vi "Remove Connection from State (SysDef).vi"(8 "error in (no error)":errorcluster, 9 "Connection":T1, 10 "State":string, 11 "Channel Ref in":T2 format="%.0x") -> (0 "error out":errorcluster, 1 "connection found":bool, 3 "Channel Ref out":T2=18446744073709551615 format="%.0x")   [LabVIEW 2017, in "Switch Scripting.lvlib"]
uses:
  Switch Scripting.lvlib
  <vilib>/NI Veristand/Custom Device API/Custom Device Item Ref.ctl
  Connection.ctl
  NationalInstruments.VeriStand.SystemDefinitionAPI
  <vilib>/NI VeriStand/Custom Device API/Custom Device API.lvlib
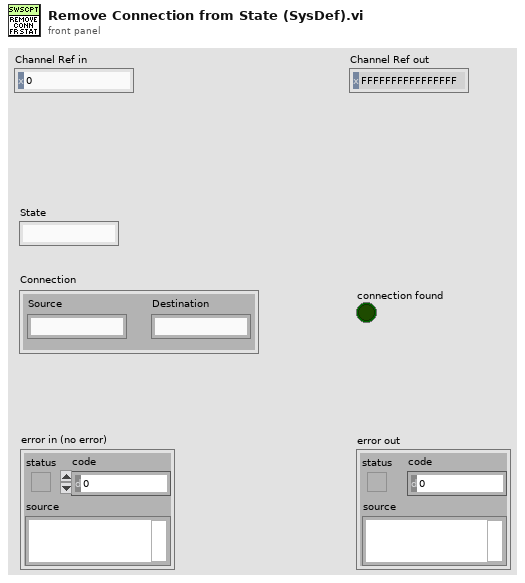
[diagram p1: front panel]
types:
  T1 = typedef "Switch Scripting.lvlib/Connection.ctl" = cluster{"Source":string, "Destination":string}
  T2 = typedef "Custom Device API.lvlib/Custom Device Item Ref.ctl" = u64
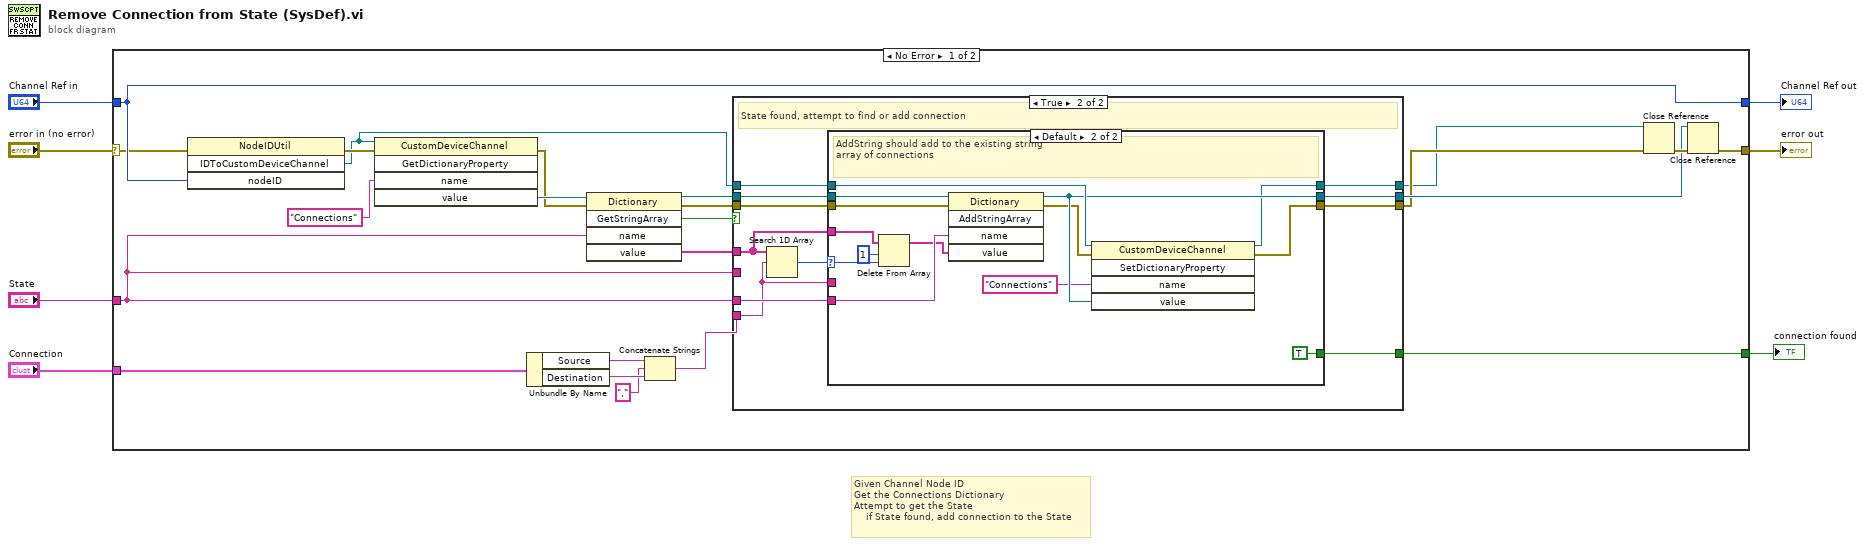
[diagram p0: block diagram]
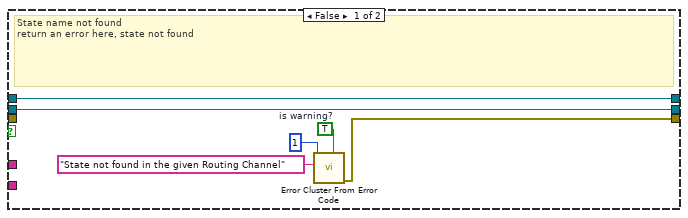
[diagram p2: hidden frame]
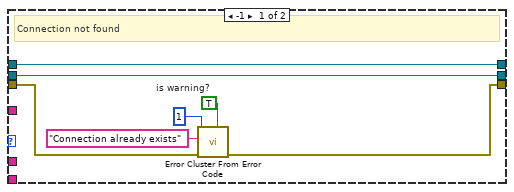
[diagram p3: hidden frame]
diagram:
  # "Given Channel Node ID\nGet the Connections Dictionary\nAttempt to get the State\n    if State found, add connection to the State"
  n1 = case shown="No Error" "error in (no error)" {
    selector: "error in (no error)" -> [w25 w70]
    tunnel: [w30 w70] -> w6
    tunnel: "Channel Ref in" -> [w26 w69]
    tunnel: [w26 w69] -> w4
    tunnel: "State" -> [w13 _]
    tunnel: "Connection" -> [w20 _]
    tunnel: [w8 _] -> w1
    frame No Error {
      n2 = invoke class="NodeIDUtil" method="IDToCustomDeviceChannel"(error in=w25, "nodeID"=w26) -> (error out=w28:errorcluster, "IDToCustomDeviceChannel"=w10:refnum<k24>)  [unwired: 2 in, 2 out]
      n3 = invoke class="CustomDeviceChannel" method="GetDictionaryProperty"(reference=w10, error in=w28, "name"="Connections") -> (error out=w22:errorcluster, "value"=w23:refnum<k24>)  [unwired: 2 in, 3 out]
      n4 = Unbundle By Name(w20) -> ("Source"=w17:string, "Destination"=w18:string)
      n5 = invoke class="Dictionary" method="GetStringArray"(reference=w23, error in=w22, "name"=w13) -> (reference out=w14:refnum<k24>, error out=w19:errorcluster, "GetStringArray"=w21:bool, "value"=w24:string[])  [unwired: 2 in, 1 out]
      n6 = Concatenate Strings(w17, "," ("string"), w18) -> (w15:string)
      n7 = case shown="True" w21 {
        tunnel: w24 -> [_ w39]
        tunnel: w19 -> [_ w46]
        tunnel: w15 -> [_ w38]
        tunnel: [w33 w45] -> w11
        tunnel: w13 -> [_ w44]
        tunnel: w14 -> [w32 w43]
        tunnel: [w32 w42] -> w12
        tunnel: w13 -> [_ _]
        tunnel: w10 -> [w31 w41]
        tunnel: [w31 w40] -> w9
        tunnel: [_ w37] -> w8
        frame False {
          w35 = TRUE  # is warning?
          # "State name not found\nreturn an error here, state not found"
          n8 = call <vilib>:"Error Cluster From Error Code.vi"("is warning? (False)"=w35, "error message (\"\")"="State not found in the given Routing Channel" ("error message (\"\")"), "error code (0)"=1) -> ("error out"=w33:errorcluster)  [unwired: 6 in]
        }
        frame True {
          # "State found, attempt to find or add connection"
          n9 = Search 1D Array(1D array=w39, element=w38) -> (index of element=w47:i32)  [unwired: 1 in]
          n10 = case shown="Default" w47 {
            selector: w47 -> [_ w59]
            tunnel: w46 -> [w51 w58]
            tunnel: [w50 w62] -> w45
            tunnel: w44 -> [_ w68]
            tunnel: w43 -> [w49 w67]
            tunnel: [w49 w65] -> w42
            tunnel: w41 -> [w48 w66]
            tunnel: [w48 w61] -> w40
            tunnel: w39 -> [_ w60]
            tunnel: w38 -> [_ _]
            tunnel: [_ TRUE] -> w37
            frame -1 {
              w53 = TRUE  # is warning?
              # "Connection not found"
              n11 = call <vilib>:"Error Cluster From Error Code.vi"("is warning? (False)"=w53, "error in (no error)"=w51, "error message (\"\")"="Connection already exists" ("error message (\"\")"), "error code (0)"=1) -> ("error out"=w50:errorcluster)  [unwired: 5 in]
            }
            frame Default {
              # "AddString should add to the existing string\narray of connections"
              n12 = Delete From Array(array=w60, length=1, index=w59) -> (array with subset deleted=w57:string[])  [unwired: 1 out]
              n13 = invoke class="Dictionary" method="AddStringArray"(reference=w67, error in=w58, "name"=w68, "value"=w57) -> (reference out=w65:refnum<k24>, error out=w63:errorcluster)  [unwired: 1 in, 3 out]
              n14 = invoke class="CustomDeviceChannel" method="SetDictionaryProperty"(reference=w66, error in=w63, "name"="Connections", "value"=w65) -> (reference out=w61:refnum<k24>, error out=w62:errorcluster)  [unwired: 1 in, 3 out]
            }
          }
        }
      }
      n15 = Close Reference(reference=w9, error in (no error)=w11) -> (error out=w29:errorcluster)
      n16 = Close Reference(reference=w12, error in (no error)=w29) -> (error out=w30:errorcluster)
    }
    frame Error {
    }
  }
  "Channel Ref out" <- w4
  "error out" <- w6
  "connection found" <- w1
